vi "Query Options.vi"(8 "error in (no error)":errorcluster, 11 "Instrument in":refnum<class "Instrument.lvclass">) -> (0 "error out":errorcluster, 2 "Options":string[](array[string]), 3 "Instrument out":refnum<class "Instrument.lvclass">)   [LabVIEW 2020, in "Instrument.lvclass"]
uses:
  Instrument.lvclass
  Instrument.lvclass/Instrument.ctl
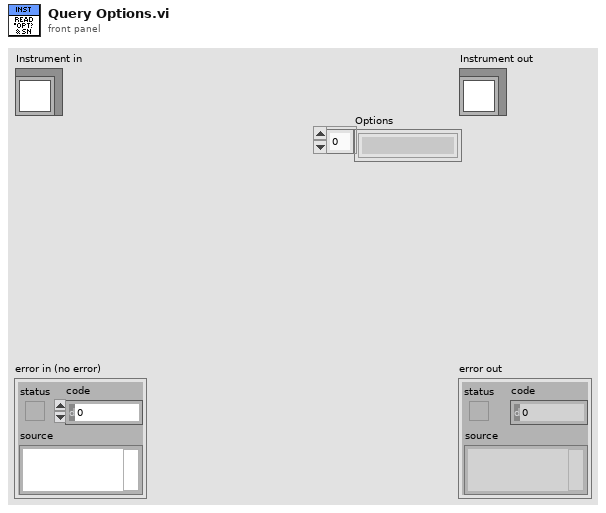
[diagram p1: front panel]
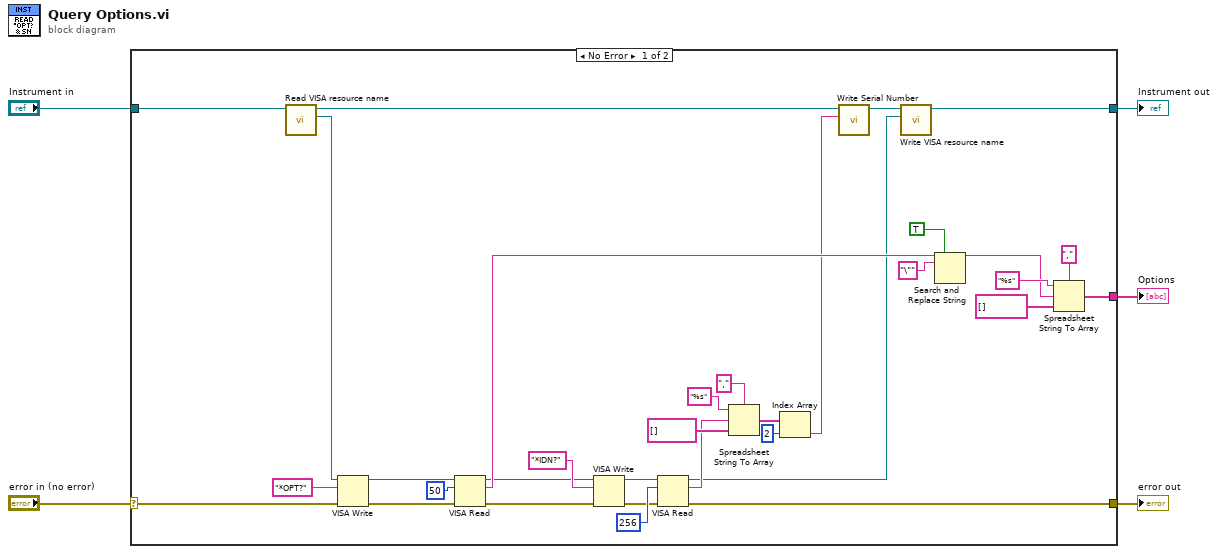
[diagram p0: block diagram]
diagram:
  n1 = case shown="No Error" "error in (no error)" {
    selector: "error in (no error)" -> [w33 w40]
    tunnel: [w8 w40] -> w4
    tunnel: [w34 w39] -> w2
    tunnel: "Instrument in" -> [w35 w39]
    tunnel: [w27 _] -> w1
    frame No Error {
      n2 = call "Read VISA resource name.vi"("Instrument in"=w35) -> ("VISA resource name"=w37:refnum<visa-resource-name>, "Instrument out"=w7:refnum<class "Instrument.lvclass">)  [unwired: 9 in]
      n3 = VISA Write(VISA resource name=w37, write buffer="*OPT?", error in (no error)=w33) -> (VISA resource name out=w36:refnum<visa-resource-name>, error out=w32:errorcluster)  [unwired: 1 out]
      n4 = VISA Read(VISA resource name=w36, byte count=u32 50, error in (no error)=w32) -> (VISA resource name out=w9:refnum<visa-resource-name>, read buffer=w24:string, error out=w11:errorcluster)  [unwired: 1 out]
      n5 = VISA Write(VISA resource name=w9, write buffer="*IDN?", error in (no error)=w11) -> (VISA resource name out=w21:refnum<visa-resource-name>, error out=w20:errorcluster)  [unwired: 1 out]
      n6 = VISA Read(VISA resource name=w21, byte count=u32 256, error in (no error)=w20) -> (VISA resource name out=w10:refnum<visa-resource-name>, read buffer=w12:string, error out=w8:errorcluster)  [unwired: 1 out]
      n7 = Spreadsheet String To Array(delimiter (Tab)=",", format string="%s", spreadsheet string=w12, array type (2D Dbl)=string[] []) -> (array=w16:string[])
      n8 = Index Array(array=w16, index=2) -> (element=w13:string)
      n9 = call-dynamic "Write Serial Number.vi"("Serial Number"=w13, "Instrument in"=w7) -> ("Instrument out"=w6:refnum<class "Instrument.lvclass">)  [unwired: 9 in]
      n10 = call "Write VISA resource name.vi"("VISA resource name"=w10, "Instrument in"=w6) -> ("Instrument out"=w34:refnum<class "Instrument.lvclass">)  [unwired: 9 in]
      n11 = Search and Replace String(replace all?=TRUE ("replace all? (F)"), input string=w24, search string="\"") -> (result string=w23:string)  [unwired: 5 in, 3 out]
      n12 = Spreadsheet String To Array(delimiter (Tab)=",", format string="%s", spreadsheet string=w23, array type (2D Dbl)=string[] []) -> (array=w27:string[])
    }
    frame Error {
    }
  }
  "error out" <- w4
  "Instrument out" <- w2
  "Options" <- w1
